vi "Table-Determine clicked cell index.vi"(8 "error in (no error)":errorcluster, 9 "Coords":T1, 11 "Table in":refnum<vi>) -> (0 "error out":errorcluster, 1 "Cell Position":T2, 2 "In Bounds?":bool, 3 "Table out":refnum<vi>)   [LabVIEW 2020]
uses:
  <vilib>/Utility/miscctls.llb/LVRowAndColumnTypeDef.ctl
  <vilib>/Utility/miscctls.llb/LVPoint32TypeDef.ctl
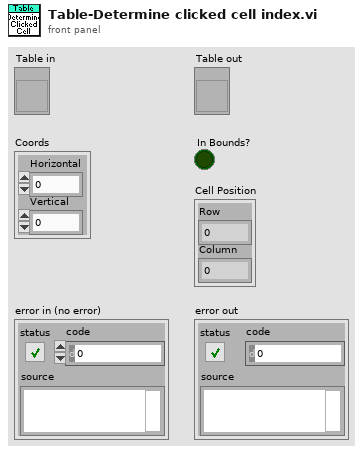
[diagram p1: front panel]
types:
  T1 = typedef "LVPoint32TypeDef.ctl" = cluster{"Horizontal":i32, "Vertical":i32}
  T2 = typedef "LVRowAndColumnTypeDef.ctl" = cluster{"Row":i32, "Column":i32}
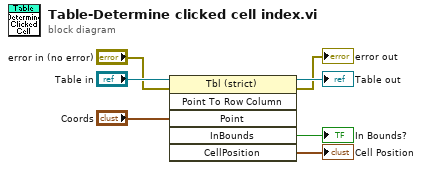
[diagram p0: block diagram]
diagram:
  n1 = invoke on="Invoke Node" class="Tbl (strict)" method="Point To Row Column"(reference="Table in", error in="error in (no error)", "Point"="Coords") -> (reference out=→"Table out":refnum<vi>, error out=→"error out":errorcluster, "InBounds"=→"In Bounds?":bool, "CellPosition"=→"Cell Position":T2)  [unwired: 3 in, 2 out]
